vi "GetParam.vi"(8 "error in (no error)":errorcluster caption="entrée d'erreur (pas d'erreur)", 11 "KFold.lvclass":refnum<class "KFold.lvclass">) -> (0 "error out":errorcluster caption="sortie d'erreur", 2 "KFold":T1={"n_splits"=5, "shuffle"=FALSE, "random_state"=-1} {"random_state" min=-1}, 3 "KFold.lvclass":refnum<class "KFold.lvclass">)   [LabVIEW 2020, in "KFold.lvclass"]
doc: "Get Parameters"
uses:
  KFold.lvclass
  KFold.lvclass/KFold.ctl
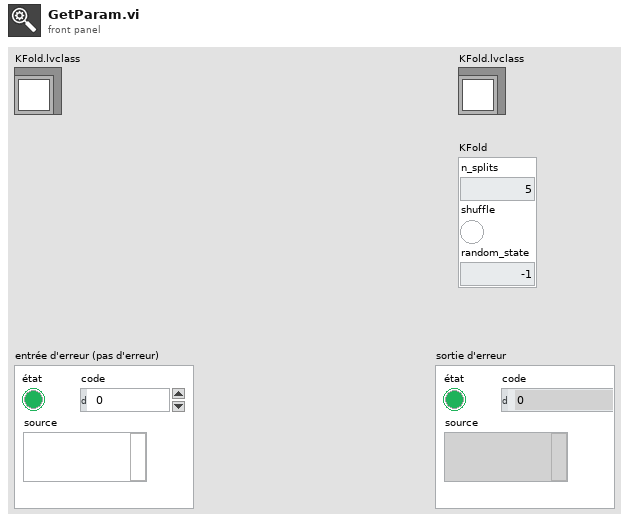
[diagram p1: front panel]
types:
  T1 = cluster{"n_splits":i32, "shuffle":bool, "random_state":i32}
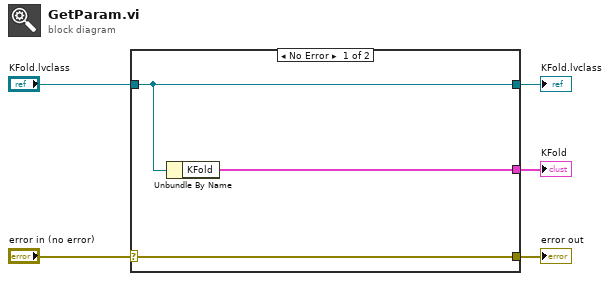
[diagram p0: block diagram]
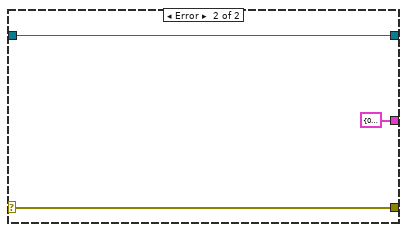
[diagram p2: hidden frame]
diagram:
  n1 = case shown="No Error" "error in (no error)" {
    selector: "error in (no error)" -> [w8 w10]
    tunnel: [w8 w10] -> w4
    tunnel: [w7 w11] -> w2
    tunnel: "KFold.lvclass" -> [w7 w11]
    tunnel: [w6 T1 {"n_splits"=0, "shuffle"=FALSE, "random_state"=0} ("KFold")] -> w1
    frame No Error {
      n2 = Unbundle By Name(w7) -> ("KFold"=w6:T1)
    }
    frame Error {
    }
  }
  "error out" <- w4
  "KFold.lvclass" <- w2
  "KFold" <- w1
